vi "Project-overflow.vi"() -> ()   [LabVIEW 2016]
uses:
  <vilib>/DAQmx/read.llb/DAQmx Read (Digital Bool 1Line 1Point).vi
  <vilib>/DAQmx/create/channels.llb/DAQmx Create Channel (DI-Digital Input).vi
  <vilib>/DAQmx/write.llb/DAQmx Write (Digital Bool 1Line 1Point).vi
  <vilib>/DAQmx/create/channels.llb/DAQmx Create Channel (DO-Digital Output).vi
  <vilib>/ptbypt/NI_PtbyPt.lvlib
panel:
  out "Laser Sensor":bool
  in  "Emergency Stop":bool
  out "Use R2":bool
  out "Use R1":bool
  out "Register Bit #1":bool
  out "Register Bit #2":bool
  out "Output Queue Counter":dbl
  out "Rejection Pusher":bool
  out "Metal Sensor 2":bool
  out "Proximity Sensor":bool
  out "Complete or not":bool
  out "Plastic In Queue":dbl
  out "Hopper":bool
  out "Pusher":bool=TRUE
  out "Plastic or not":bool
  out "Belt 2":bool=TRUE
  out "Belt 1":bool=TRUE
  out "Stoped":bool=TRUE
  out "Started":bool=TRUE
  in  "PAUSE":bool
  in  "OFF":bool
  in  "ON":bool
  out "Rejected Pieces":dbl
  out "Completed Pieces":dbl
  out "Don't Push?":bool
  out "Is there anything there?":bool
  # "Main Control"
  # "Sorting Station"
  # "QA Sorting Station"
  # "QA Sorting Register Value"
  # "Result Counter"
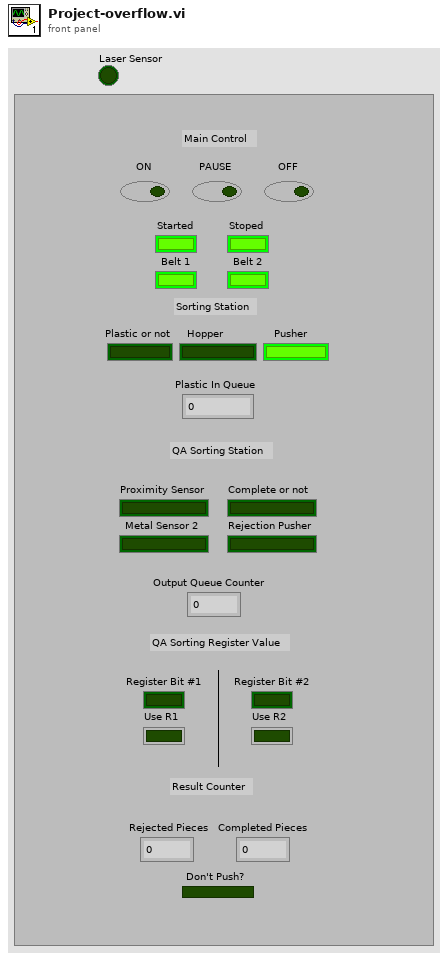
[diagram p1: front panel]
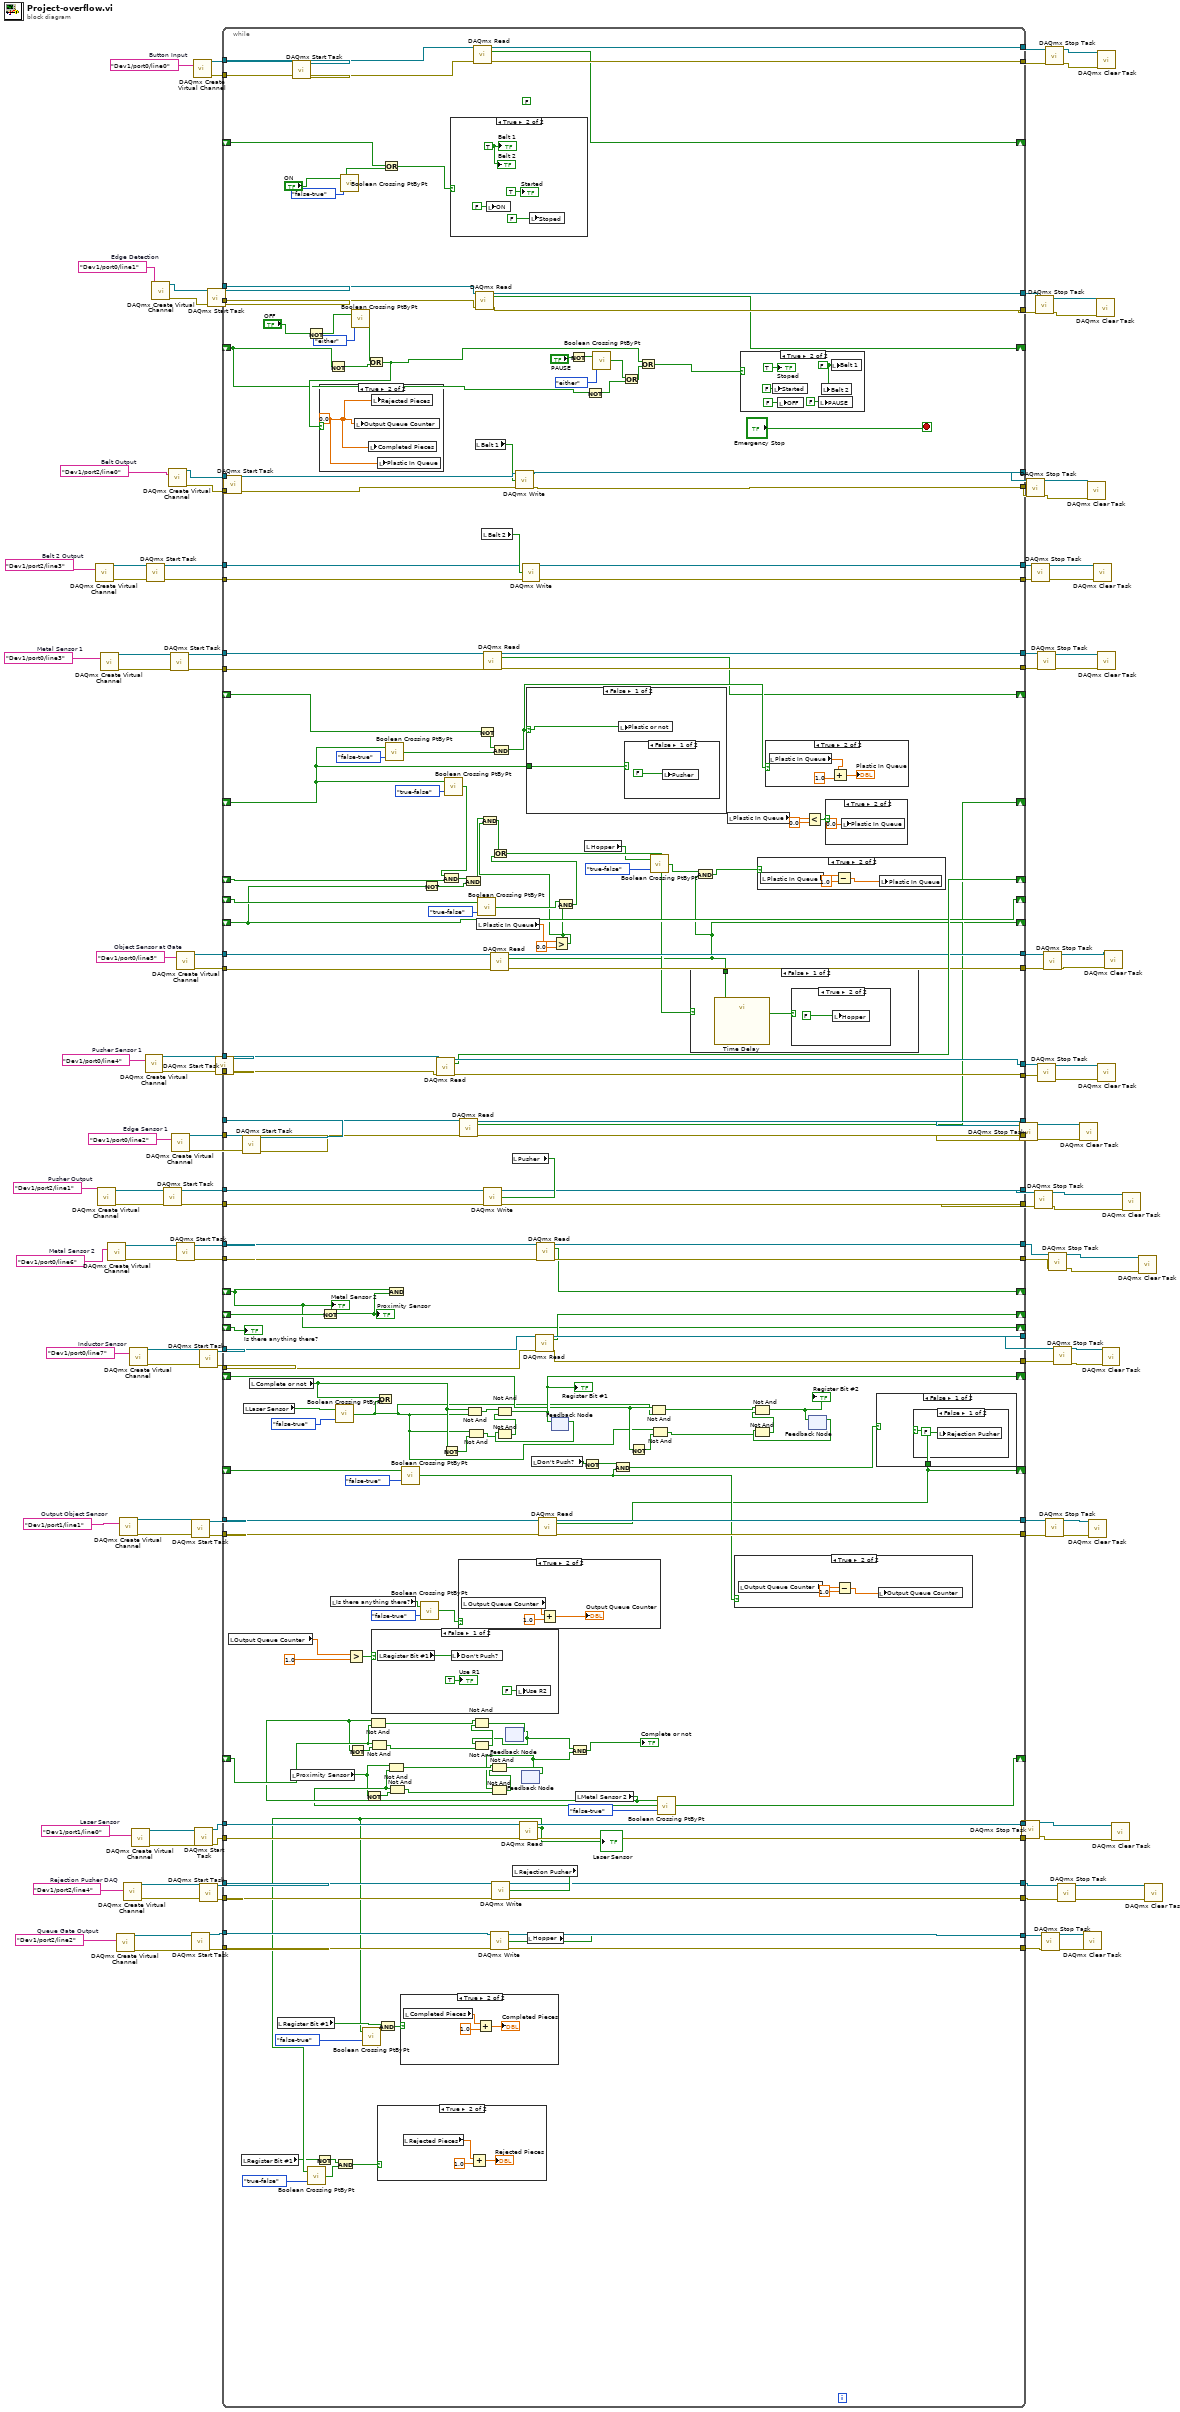
[diagram p0: block diagram]
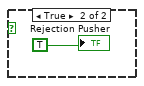
[diagram p3: hidden frame]
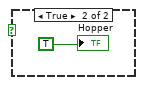
[diagram p5: hidden frame]
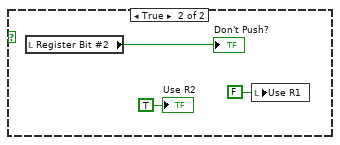
[diagram p12: hidden frame]
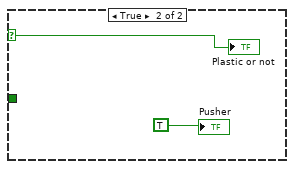
[diagram p16: hidden frame]
diagram:
  w5 = tag "Dev1/port0/line5"  # Object Sensor at Gate
  w12 = tag "Dev1/port1/line0"  # Laser Sensor
  w25 = tag "Dev1/port0/line7"  # Inductor Sensor
  w28 = tag "Dev1/port1/line1"  # Output Object Sensor
  w43 = tag "Dev1/port0/line6"  # Metal Sensor 2
  w46 = tag "Dev1/port2/line4"  # Rejection Pusher DAQ
  w57 = tag "Dev1/port2/line2"  # Queue Gate Output
  w64 = tag "Dev1/port2/line3"  # Belt 2 Output
  w75 = tag "Dev1/port0/line4"  # Pusher Sensor 1
  w84 = tag "Dev1/port0/line2"  # Edge Sensor 1
  w89 = tag "Dev1/port2/line1"  # Pusher Output
  w90 = tag "Dev1/port0/line1"  # Edge Detection
  w91 = tag "Dev1/port0/line0"  # Button Input
  w92 = tag "Dev1/port0/line3"  # Metal Sensor 1
  w93 = tag "Dev1/port2/line0"  # Belt Output
  n1 = call-poly <vilib>:"DAQmx Create Virtual Channel.vi"("lines"=w64) -> ("task out"=w66:refnum<k21>, "error out"=w65:errorcluster)  [unwired: 13 in]
  n2 = call-poly <vilib>:"DAQmx Create Virtual Channel.vi"("lines"=w89) -> ("task out"=w101:refnum<k21>, "error out"=w100:errorcluster)  [unwired: 13 in]
  n3 = call-poly <vilib>:"DAQmx Create Virtual Channel.vi"("lines"=w92) -> ("task out"=w109:refnum<k21>, "error out"=w108:errorcluster)  [unwired: 13 in]
  n4 = call-poly <vilib>:"DAQmx Create Virtual Channel.vi"("lines"=w43) -> ("task out"=w45:refnum<k21>, "error out"=w44:errorcluster)  [unwired: 13 in]
  n5 = call-poly <vilib>:"DAQmx Create Virtual Channel.vi"("lines"=w57) -> ("task out"=w59:refnum<k21>, "error out"=w58:errorcluster)  [unwired: 13 in]
  n6 = call-poly <vilib>:"DAQmx Create Virtual Channel.vi"("lines"=w28) -> ("task out"=w30:refnum<k21>, "error out"=w29:errorcluster)  [unwired: 13 in]
  n7 = call-poly <vilib>:"DAQmx Create Virtual Channel.vi"("lines"=w46) -> ("task out"=w48:refnum<k21>, "error out"=w47:errorcluster)  [unwired: 13 in]
  n8 = call-poly <vilib>:"DAQmx Create Virtual Channel.vi"("lines"=w25) -> ("task out"=w27:refnum<k21>, "error out"=w26:errorcluster)  [unwired: 13 in]
  n9 = call-poly <vilib>:"DAQmx Create Virtual Channel.vi"("lines"=w12) -> ("task out"=w14:refnum<k21>, "error out"=w13:errorcluster)  [unwired: 13 in]
  n10 = call-poly <vilib>:"DAQmx Create Virtual Channel.vi"("lines"=w75) -> ("task out"=w77:refnum<k21>, "error out"=w76:errorcluster)  [unwired: 13 in]
  n11 = call <vilib>:"DAQmx Start Task.vi"("task/channels in"=w66, "error in"=w65) -> ("task out"=w63:refnum<k21>, "error out"=w62:errorcluster)  [unwired: 12 in]
  n12 = call-poly <vilib>:"DAQmx Create Virtual Channel.vi"("lines"=w90) -> ("task out"=w125:refnum<k21>, "error out"=w124:errorcluster)  [unwired: 13 in]
  n13 = call <vilib>:"DAQmx Start Task.vi"("task/channels in"=w101, "error in"=w100) -> ("task out"=w95:refnum<k21>, "error out"=w94:errorcluster)  [unwired: 12 in]
  n14 = call-poly <vilib>:"DAQmx Create Virtual Channel.vi"("lines"=w93) -> ("task out"=w113:refnum<k21>, "error out"=w112:errorcluster)  [unwired: 13 in]
  n15 = call <vilib>:"DAQmx Start Task.vi"("task/channels in"=w109, "error in"=w108) -> ("task out"=w107:refnum<k21>, "error out"=w106:errorcluster)  [unwired: 12 in]
  n16 = call-poly <vilib>:"DAQmx Create Virtual Channel.vi"("lines"=w84) -> ("task out"=w86:refnum<k21>, "error out"=w85:errorcluster)  [unwired: 13 in]
  n17 = call <vilib>:"DAQmx Start Task.vi"("task/channels in"=w45, "error in"=w44) -> ("task out"=w40:refnum<k21>, "error out"=w39:errorcluster)  [unwired: 12 in]
  n18 = call-poly <vilib>:"DAQmx Create Virtual Channel.vi"("lines"=w5) -> ("task out"=w4:refnum<k21>, "error out"=w3:errorcluster)  [unwired: 13 in]
  n19 = call <vilib>:"DAQmx Start Task.vi"("task/channels in"=w30, "error in"=w29) -> ("task out"=w24:refnum<k21>, "error out"=w23:errorcluster)  [unwired: 12 in]
  n20 = call <vilib>:"DAQmx Start Task.vi"("task/channels in"=w59, "error in"=w58) -> ("task out"=w56:refnum<k21>, "error out"=w55:errorcluster)  [unwired: 12 in]
  n21 = call-poly <vilib>:"DAQmx Create Virtual Channel.vi"("lines"=w91) -> ("task out"=w133:refnum<k21>, "error out"=w132:errorcluster)  [unwired: 13 in]
  n22 = call <vilib>:"DAQmx Start Task.vi"("task/channels in"=w14, "error in"=w13) -> ("task out"=w11:refnum<k21>, "error out"=w8:errorcluster)  [unwired: 12 in]
  n23 = call <vilib>:"DAQmx Start Task.vi"("task/channels in"=w27, "error in"=w26) -> ("task out"=w22:refnum<k21>, "error out"=w21:errorcluster)  [unwired: 12 in]
  n24 = call <vilib>:"DAQmx Start Task.vi"("task/channels in"=w48, "error in"=w47) -> ("task out"=w38:refnum<k21>, "error out"=w37:errorcluster)  [unwired: 12 in]
  n25 = call <vilib>:"DAQmx Start Task.vi"("task/channels in"=w125, "error in"=w124) -> ("task out"=w122:refnum<k21>, "error out"=w123:errorcluster)  [unwired: 12 in]
  n26 = call <vilib>:"DAQmx Start Task.vi"("task/channels in"=w77, "error in"=w76) -> ("task out"=w74:refnum<k21>, "error out"=w73:errorcluster)  [unwired: 12 in]
  n27 = call <vilib>:"DAQmx Start Task.vi"("task/channels in"=w113, "error in"=w112) -> ("task out"=w111:refnum<k21>, "error out"=w110:errorcluster)  [unwired: 12 in]
  n28 = call <vilib>:"DAQmx Start Task.vi"("task/channels in"=w86, "error in"=w85) -> ("task out"=w83:refnum<k21>, "error out"=w82:errorcluster)  [unwired: 12 in]
  n29 = call <vilib>:"DAQmx Start Task.vi"("task/channels in"=w133, "error in"=w132) -> ("task out"=w131:refnum<k21>, "error out"=w130:errorcluster)  [unwired: 12 in]
  n30 = while {
    tunnel: w131 -> [w317]
    tunnel: w130 -> [w316]
    tunnel: [w315] -> w129
    tunnel: [w314] -> w128
    shift-right: [w312] -> _
    shift-left: _ -> [w246]
    tunnel: w123 -> [w311]
    tunnel: w122 -> [w310]
    tunnel: [w309] -> w121
    tunnel: [w308] -> w118
    shift-right: [w307] -> _
    shift-left: _ -> [w184]
    tunnel: [w306] -> w115
    tunnel: [w303] -> w114
    tunnel: w111 -> [w305]
    tunnel: w110 -> [w304]
    tunnel: w107 -> [w301]
    tunnel: w106 -> [w300]
    tunnel: [w299] -> w103
    tunnel: [w298] -> w102
    shift-right: [w157] -> _
    shift-left: _ -> [w156]
    tunnel: [w296] -> w97
    tunnel: [w295] -> w96
    tunnel: w95 -> [w294]
    tunnel: w94 -> [w293]
    tunnel: w83 -> [w292]
    tunnel: w82 -> [w291]
    tunnel: [w290] -> w81
    tunnel: [w289] -> w80
    shift-right: [w159] -> _
    shift-left: _ -> [w152]
    tunnel: w74 -> [w287]
    tunnel: w73 -> [w286]
    tunnel: [w285] -> w72
    tunnel: [w284] -> w71
    tunnel: [w281] -> w68
    tunnel: [w280] -> w67
    tunnel: w63 -> [w279]
    tunnel: w62 -> [w278]
    tunnel: w56 -> [w277]
    tunnel: w55 -> [w276]
    tunnel: [w275] -> w54
    tunnel: [w274] -> w53
    shift-right: [w272] -> _
    shift-left: _ -> [w271]
    tunnel: [w267] -> w42
    tunnel: [w266] -> w41
    tunnel: w40 -> [w265]
    tunnel: w39 -> [w264]
    tunnel: w38 -> [w263]
    tunnel: w37 -> [w262]
    tunnel: [w261] -> w36
    tunnel: [w260] -> w35
    shift-right: [w259] -> _
    shift-left: _ -> [w212]
    tunnel: w24 -> [w258]
    tunnel: w23 -> [w257]
    tunnel: w22 -> [w256]
    tunnel: w21 -> [w255]
    tunnel: [w254] -> w20
    tunnel: [w253] -> w19
    tunnel: [w252] -> w18
    tunnel: [w251] -> w17
    shift-right: [w160] -> _
    shift-left: _ -> [w234]
    shift-right: [w250] -> _
    shift-left: _ -> [w249]
    shift-right: [w212] -> _
    shift-left: _ -> [w236]
    tunnel: w11 -> [w232]
    tunnel: [w231] -> w10
    tunnel: [w230] -> w9
    tunnel: w8 -> [w229]
    shift-right: [w214] -> _
    shift-left: _ -> [w213]
    tunnel: w4 -> [w183]
    tunnel: w3 -> [w182]
    tunnel: [w181] -> w2
    tunnel: [w180] -> w1
    shift-right: [w154] -> _
    shift-left: _ -> [w175]
    shift-right: [w175] -> _
    shift-left: _ -> [w178]
    shift-right: [w138] -> _
    shift-left: _ -> [w145]
    stop <- "Emergency Stop" stop-if-true
    (unwired) FALSE ("Boolean")
    n31 = local read "Output Queue Counter"() -> (w222:dbl)
    n32 = local read "Register Bit #1"() -> (w193:bool)
    n33 = local read "Laser Sensor"() -> (w237:bool)
    n34 = local read "Complete or not"() -> (w211:bool)
    n35 = local read "Register Bit #1"() -> (w200:bool)
    n36 = local read "Proximity Sensor"() -> (w137:bool)
    n37 = Not(x="OFF") -> (.not. x?=w206:bool)
    n38 = Not(x=w193) -> (.not. x?=w194:bool)
    n39 = Not(x=w249) -> (.not. x?=w244:bool)
    "Proximity Sensor" <- w244
    n40 = Not(x=w184) -> (.not. x?=w245:bool)
    n41 = local read "Is there anything there?"() -> (w226:bool)
    n42 = call <vilib>:"Boolean Crossing PtByPt.vi"("direction"=enum16{"either", "false-true", "true-false"}."false-true", "input"=w237) -> ("crossing"=w210:bool)  [unwired: 1 in]
    n43 = call <vilib>:"Boolean Crossing PtByPt.vi"("direction"=enum16{"either", "false-true", "true-false"}."false-true", "input"="ON") -> ("crossing"=w209:bool)  [unwired: 1 in]
    n44 = Greater?(x=w222, y=1.0) -> (0:w221:bool)
    n45 = call <vilib>:"Boolean Crossing PtByPt.vi"("direction"=enum16{"either", "false-true", "true-false"}."either", "input"=w206) -> ("crossing"=w207:bool)  [unwired: 1 in]
    n46 = Not(x=w137) -> (.not. x?=w140:bool)
    n47 = Or(x=w207, y=w245) -> (x .or. y?=w185:bool)
    n48 = case shown="True" w185 {
      frame False {
      }
      frame True {
        w331 = 0.0 ("Completed Piece")
        n49 = local write "Output Queue Counter"(w331) -> ()
        n50 = local write "Completed Pieces"(w331) -> ()
        n51 = local write "Rejected Pieces"(w331) -> ()
        n52 = local write "Plastic In Queue"(w331) -> ()
      }
    }
    n53 = case shown="False" w221 {
      frame False {
        n54 = local read "Register Bit #1"() -> (w340:bool)
        n55 = local write "Don't Push?"(w340) -> ()
        n56 = local write "Use R2"(FALSE ("Use R2")) -> ()
        "Use R1" <- TRUE ("Use R1")
      }
      frame True {
        n57 = local read "Register Bit #2"() -> (→"Don't Push?":bool)
        n58 = local write "Use R1"(FALSE ("Use R1")) -> ()
        "Use R2" <- TRUE ("Use R2")
      }
    }
    n59 = Or(x=w211, y=w210) -> ()  [unwired: 1 out]
    n60 = Or(x=w246, y=w209) -> (x .or. y?=w247:bool)
    n61 = call <vilib>:"Boolean Crossing PtByPt.vi"("direction"=enum16{"either", "false-true", "true-false"}."false-true", "input"=w152) -> ("crossing"=w273:bool)  [unwired: 1 in]
    n62 = And(x=w212, y=w244) -> ()  [unwired: 1 out]
    n63 = call <vilib>:"Boolean Crossing PtByPt.vi"("direction"=enum16{"either", "false-true", "true-false"}."false-true", "input"=w234) -> ("crossing"=w224:bool)  [unwired: 1 in]
    n64 = call <vilib>:"Boolean Crossing PtByPt.vi"("direction"=enum16{"either", "false-true", "true-false"}."false-true", "input"=w226) -> ("crossing"=w227:bool)  [unwired: 1 in]
    n65 = Not(x=w175) -> (.not. x?=w176:bool)
    n66 = call-poly <vilib>:"DAQmx Read.vi"("task/channels in"=w287, "error in"=w286) -> ("task out"=w284:refnum<k21>, "data"=w272:bool, "error out"=w285:errorcluster)  [unwired: 11 in]
    n67 = Not(x=w211) -> (.not. x?=w239:bool)
    n68 = call <vilib>:"Boolean Crossing PtByPt.vi"("direction"=enum16{"either", "false-true", "true-false"}."true-false", "input"=w152) -> ("crossing"=w269:bool)  [unwired: 1 in]
    n69 = And(x=w269, y=w271) -> (x .and. y?=w177:bool)
    n70 = case shown="True" w247 {
      frame False {
      }
      frame True {
        w361 = TRUE
        n71 = local write "ON"(FALSE ("ON")) -> ()
        n72 = local write "Stoped"(FALSE) -> ()
        "Started" <- TRUE ("Boolean")
        "Belt 1" <- w361
        "Belt 2" <- w361
      }
    }
    n73 = case shown="True" w227 {
      frame False {
      }
      frame True {
        n74 = local read "Output Queue Counter"() -> (w347:dbl)
        n75 = Add(x=w347, y=1.0) -> (x+y=→"Output Queue Counter":dbl)
      }
    }
    n76 = call-poly <vilib>:"DAQmx Read.vi"("task/channels in"=w292, "error in"=w291) -> ("task out"=w289:refnum<k21>, "data"=w159:bool, "error out"=w290:errorcluster)  [unwired: 11 in]
    n77 = And(x=w177, y=w176) -> (x .and. y?=w169:bool)
    n78 = Not And(1:w210, 2:w211) -> (0:w240:bool)
    n79 = Not And(1:w239, 2:w210) -> (0:w241:bool)
    n80 = call-poly <vilib>:"DAQmx Read.vi"("task/channels in"=w317, "error in"=w316) -> ("task out"=w315:refnum<k21>, "data"=w312:bool, "error out"=w314:errorcluster)  [unwired: 11 in]
    n81 = call-poly <vilib>:"DAQmx Read.vi"("task/channels in"=w310, "error in"=w311) -> ("task out"=w309:refnum<k21>, "data"=w307:bool, "error out"=w308:errorcluster)  [unwired: 11 in]
    n82 = local read "Belt 1"() -> (w302:bool)
    n83 = local read "Plastic In Queue"() -> (w173:dbl)
    n84 = call <vilib>:"Boolean Crossing PtByPt.vi"("direction"=enum16{"either", "false-true", "true-false"}."true-false", "input"=w178) -> ("crossing"=w171:bool)  [unwired: 1 in]
    n85 = Not(x=w156) -> (.not. x?=w288:bool)
    n86 = local read "Belt 2"() -> (w282:bool)
    n87 = call-poly <vilib>:"DAQmx Read.vi"("task/channels in"=w301, "error in"=w300) -> ("task out"=w299:refnum<k21>, "data"=w157:bool, "error out"=w298:errorcluster)  [unwired: 11 in]
    n88 = call-poly <vilib>:"DAQmx Read.vi"("task/channels in"=w183, "error in"=w182) -> ("task out"=w181:refnum<k21>, "data"=w154:bool, "error out"=w180:errorcluster)  [unwired: 11 in]
    n89 = And(x=w288, y=w273) -> (x .and. y?=w174:bool)
    n90 = feedback #1() -> (w136:bool)  [unwired: 1 in]
    n91 = local read "Pusher"() -> (w297:bool)
    n92 = call-poly <vilib>:"DAQmx Write.vi"("task/channels in"=w294, "data"=w297, "error in"=w293) -> ("task out"=w296:refnum<k21>, "error out"=w295:errorcluster)  [unwired: 10 in, 1 out]
    n93 = local read "Rejection Pusher"() -> (w268:bool)
    n94 = call-poly <vilib>:"DAQmx Write.vi"("task/channels in"=w263, "data"=w268, "error in"=w262) -> ("task out"=w261:refnum<k21>, "error out"=w260:errorcluster)  [unwired: 10 in, 1 out]
    n95 = call-poly <vilib>:"DAQmx Write.vi"("task/channels in"=w305, "data"=w302, "error in"=w304) -> ("task out"=w306:refnum<k21>, "error out"=w303:errorcluster)  [unwired: 10 in, 1 out]
    n96 = call-poly <vilib>:"DAQmx Read.vi"("task/channels in"=w232, "error in"=w229) -> ("task out"=w231:refnum<k21>, "data"=w197:bool, "error out"=w230:errorcluster)  [unwired: 11 in]
    "Laser Sensor" <- w197
    n97 = call <vilib>:"Boolean Crossing PtByPt.vi"("direction"=enum16{"either", "false-true", "true-false"}."true-false", "input"=w197) -> ("crossing"=w195:bool)  [unwired: 1 in]
    n98 = And(x=w194, y=w195) -> (x .and. y?=w196:bool)
    n99 = call <vilib>:"Boolean Crossing PtByPt.vi"("direction"=enum16{"either", "false-true", "true-false"}."false-true", "input"=w197) -> ("crossing"=w199:bool)  [unwired: 1 in]
    n100 = case shown="True" w196 {
      frame False {
      }
      frame True {
        n101 = local read "Rejected Pieces"() -> (w333:dbl)
        n102 = Add(x=w333, y=1.0) -> (x+y=→"Rejected Pieces":dbl)
      }
    }
    n103 = And(x=w200, y=w199) -> (x .and. y?=w198:bool)
    n104 = case shown="True" w198 {
      frame False {
      }
      frame True {
        n105 = local read "Completed Pieces"() -> (w335:dbl)
        n106 = Add(x=w335, y=1.0) -> (x+y=→"Completed Pieces":dbl)
      }
    }
    n107 = feedback #2() -> (w135:bool)  [unwired: 1 in]
    n108 = call-poly <vilib>:"DAQmx Write.vi"("task/channels in"=w279, "data"=w282, "error in"=w278) -> ("task out"=w281:refnum<k21>, "error out"=w280:errorcluster)  [unwired: 10 in, 1 out]
    n109 = case shown="False" w174 {
      selector: w174 -> [w351 w354]
      tunnel: w152 -> [w350 _]
      frame False {
        n110 = local write "Plastic or not"(w351) -> ()
        n111 = case shown="False" w350 {
          frame False {
            n112 = local write "Pusher"(FALSE) -> ()
          }
          frame True {
          }
        }
      }
      frame True {
        "Plastic or not" <- w354
        "Pusher" <- TRUE
      }
    }
    n113 = local read "Hopper"() -> (w248:bool)
    n114 = call-poly <vilib>:"DAQmx Write.vi"("task/channels in"=w277, "data"=w248, "error in"=w276) -> ("task out"=w275:refnum<k21>, "error out"=w274:errorcluster)  [unwired: 10 in, 1 out]
    n115 = local read "Don't Push?"() -> (w228:bool)
    n116 = call-poly <vilib>:"DAQmx Read.vi"("task/channels in"=w256, "error in"=w255) -> ("task out"=w251:refnum<k21>, "data"=w250:bool, "error out"=w252:errorcluster)  [unwired: 11 in]
    n117 = call-poly <vilib>:"DAQmx Read.vi"("task/channels in"=w265, "error in"=w264) -> ("task out"=w267:refnum<k21>, "data"=w259:bool, "error out"=w266:errorcluster)  [unwired: 11 in]
    n118 = call-poly <vilib>:"DAQmx Read.vi"("task/channels in"=w258, "error in"=w257) -> ("task out"=w254:refnum<k21>, "data"=w160:bool, "error out"=w253:errorcluster)  [unwired: 11 in]
    n119 = feedback #3() -> (w242:bool)  [unwired: 1 in]
    n120 = Not And(1:w241, 2:w242) -> (0:w243:bool)
    n121 = Not And(1:w243, 2:w240) -> (0:w214:bool)
    "Register Bit #1" <- w214
    n122 = feedback-in #3(w214) -> ()
    n123 = Greater?(x=w173, y=0.0) -> (0:w168:bool)
    n124 = And(x=w169, y=w168) -> (x .and. y?=w164:bool)
    n125 = And(x=w171, y=w168) -> (x .and. y?=w163:bool)
    n126 = Or(x=w164, y=w163) -> (x .or. y?=w162:bool)
    n127 = Not(x="PAUSE") -> (.not. x?=w190:bool)
    n128 = And(x=w136, y=w135) -> (x .and. y?=→"Complete or not":bool)
    n129 = local read "Metal Sensor 2"() -> (w144:bool)
    n130 = Not(x=w144) -> (.not. x?=w148:bool)
    n131 = Not And(1:w145, 2:w144) -> (0:w149:bool)
    n132 = Not And(1:w148, 2:w145) -> (0:w150:bool)
    n133 = Not And(1:w150, 2:w136) -> (0:w151:bool)
    n134 = Not And(1:w151, 2:w149) -> (0:w147:bool)
    n135 = feedback-in #1(w147) -> ()
    n136 = Not(x=w228) -> (.not. x?=w235:bool)
    n137 = local read "Hopper"() -> (w158:bool)
    n138 = Not(x=w184) -> (.not. x?=w192:bool)
    n139 = call <vilib>:"Boolean Crossing PtByPt.vi"("direction"=enum16{"either", "false-true", "true-false"}."either", "input"=w190) -> ("crossing"=w191:bool)  [unwired: 1 in]
    n140 = And(x=w235, y=w224) -> (x .and. y?=w161:bool)
    n141 = Or(x=w191, y=w192) -> (x .or. y?=w186:bool)
    n142 = Not(x=w213) -> (.not. x?=w216:bool)
    n143 = Or(x=w185, y=w186) -> (x .or. y?=w187:bool)
    n144 = call <vilib>:"Boolean Crossing PtByPt.vi"("direction"=enum16{"either", "false-true", "true-false"}."true-false", "input"=w158) -> ("crossing"=w155:bool)  [unwired: 1 in]
    n145 = Not And(1:w210, 2:w213) -> (0:w217:bool)
    n146 = Not And(1:w216, 2:w210) -> (0:w218:bool)
    n147 = call <vilib>:"Boolean Crossing PtByPt.vi"("direction"=enum16{"either", "false-true", "true-false"}."false-true", "input"=w144) -> ("crossing"=w138:bool)  [unwired: 1 in]
    n148 = Not And(1:w138, 2:w137) -> (0:w141:bool)
    n149 = Not And(1:w140, 2:w138) -> (0:w142:bool)
    n150 = Not And(1:w142, 2:w135) -> (0:w143:bool)
    n151 = Not And(1:w143, 2:w141) -> (0:w139:bool)
    n152 = feedback-in #2(w139) -> ()
    n153 = case shown="False" w162 {
      tunnel: w154 -> [w321 _]
      frame False {
        n154 = call "Time Delay"() -> ()  [unwired: 11 in, 1 out]
        n155 = case shown="True" w321 {
          frame False {
          }
          frame True {
            n156 = local write "Hopper"(FALSE) -> ()
          }
        }
      }
      frame True {
        "Hopper" <- TRUE
      }
    }
    n157 = And(x=w155, y=w154) -> (x .and. y?=w153:bool)
    n158 = local read "Plastic In Queue"() -> (w167:dbl)
    n159 = case shown="True" w224 {
      frame False {
      }
      frame True {
        n160 = local read "Output Queue Counter"() -> (w346:dbl)
        n161 = Subtract(x=w346, y=1.0) -> (x-y=w344:dbl)
        n162 = local write "Output Queue Counter"(w344) -> ()
      }
    }
    n163 = case shown="True" w187 {
      frame False {
      }
      frame True {
        w357 = FALSE
        n164 = local write "Started"(FALSE ("Stop")) -> ()
        n165 = local write "OFF"(FALSE ("OFF")) -> ()
        n166 = local write "PAUSE"(FALSE ("Pause")) -> ()
        n167 = local write "Belt 2"(w357) -> ()
        n168 = local write "Belt 1"(w357) -> ()
        "Stoped" <- TRUE
      }
    }
    n169 = case shown="True" w153 {
      frame False {
      }
      frame True {
        n170 = local read "Plastic In Queue"() -> (w326:dbl)
        n171 = Subtract(x=w326, y=1.0) -> (x-y=w327:dbl)
        n172 = local write "Plastic In Queue"(w327) -> ()
      }
    }
    n173 = case shown="True" w174 {
      frame False {
      }
      frame True {
        n174 = local read "Plastic In Queue"() -> (w328:dbl)
        n175 = Add(x=w328, y=1.0) -> (x+y=→"Plastic In Queue":dbl)
      }
    }
    n176 = Less?(x=w167, y=0.0) -> (x < y?=w165:bool)
    n177 = feedback #4() -> (w219:bool)  [unwired: 1 in]
    n178 = Not And(1:w218, 2:w219) -> (0:w220:bool)
    n179 = Not And(1:w220, 2:w217) -> (0:w215:bool)
    "Register Bit #2" <- w215
    n180 = feedback-in #4(w215) -> ()
    n181 = case shown="True" w165 {
      frame False {
      }
      frame True {
        n182 = local write "Plastic In Queue"(0.0 ("Plastic In Queue")) -> ()
      }
    }
    n183 = case shown="False" w161 {
      tunnel: w160 -> [w318 _]
      frame False {
        n184 = case shown="False" w318 {
          frame False {
            n185 = local write "Rejection Pusher"(FALSE) -> ()
          }
          frame True {
          }
        }
      }
      frame True {
        "Rejection Pusher" <- TRUE
      }
    }
    "Metal Sensor 2" <- w212
    "Is there anything there?" <- w236
  }
  n186 = call <vilib>:"DAQmx Stop Task.vi"("task/channels in"=w80, "error in"=w81) -> ("task out"=w88:refnum<k21>, "error out"=w87:errorcluster)  [unwired: 12 in]
  n187 = call <vilib>:"DAQmx Stop Task.vi"("task/channels in"=w10, "error in"=w9) -> ("task out"=w16:refnum<k21>, "error out"=w15:errorcluster)  [unwired: 12 in]
  n188 = call <vilib>:"DAQmx Stop Task.vi"("task/channels in"=w115, "error in"=w114) -> ("task out"=w117:refnum<k21>, "error out"=w116:errorcluster)  [unwired: 12 in]
  n189 = call <vilib>:"DAQmx Stop Task.vi"("task/channels in"=w68, "error in"=w67) -> ("task out"=w70:refnum<k21>, "error out"=w69:errorcluster)  [unwired: 12 in]
  n190 = call <vilib>:"DAQmx Stop Task.vi"("task/channels in"=w97, "error in"=w96) -> ("task out"=w99:refnum<k21>, "error out"=w98:errorcluster)  [unwired: 12 in]
  n191 = call <vilib>:"DAQmx Stop Task.vi"("task/channels in"=w121, "error in"=w118) -> ("task out"=w120:refnum<k21>, "error out"=w119:errorcluster)  [unwired: 12 in]
  n192 = call <vilib>:"DAQmx Stop Task.vi"("task/channels in"=w103, "error in"=w102) -> ("task out"=w105:refnum<k21>, "error out"=w104:errorcluster)  [unwired: 12 in]
  n193 = call <vilib>:"DAQmx Stop Task.vi"("task/channels in"=w71, "error in"=w72) -> ("task out"=w79:refnum<k21>, "error out"=w78:errorcluster)  [unwired: 12 in]
  n194 = call <vilib>:"DAQmx Stop Task.vi"("task/channels in"=w54, "error in"=w53) -> ("task out"=w61:refnum<k21>, "error out"=w60:errorcluster)  [unwired: 12 in]
  n195 = call <vilib>:"DAQmx Stop Task.vi"("task/channels in"=w2, "error in"=w1) -> ("task out"=w7:refnum<k21>, "error out"=w6:errorcluster)  [unwired: 12 in]
  n196 = call <vilib>:"DAQmx Stop Task.vi"("task/channels in"=w20, "error in"=w19) -> ("task out"=w34:refnum<k21>, "error out"=w33:errorcluster)  [unwired: 12 in]
  n197 = call <vilib>:"DAQmx Stop Task.vi"("task/channels in"=w129, "error in"=w128) -> ("task out"=w126:refnum<k21>, "error out"=w127:errorcluster)  [unwired: 12 in]
  n198 = call <vilib>:"DAQmx Stop Task.vi"("task/channels in"=w42, "error in"=w41) -> ("task out"=w50:refnum<k21>, "error out"=w49:errorcluster)  [unwired: 12 in]
  n199 = call <vilib>:"DAQmx Stop Task.vi"("task/channels in"=w17, "error in"=w18) -> ("task out"=w32:refnum<k21>, "error out"=w31:errorcluster)  [unwired: 12 in]
  n200 = call <vilib>:"DAQmx Stop Task.vi"("task/channels in"=w36, "error in"=w35) -> ("task out"=w52:refnum<k21>, "error out"=w51:errorcluster)  [unwired: 12 in]
  n201 = call <vilib>:"DAQmx Clear Task.vi"("task in"=w88, "error in"=w87) -> ()  [unwired: 13 in, 1 out]
  n202 = call <vilib>:"DAQmx Clear Task.vi"("task in"=w61, "error in"=w60) -> ()  [unwired: 13 in, 1 out]
  n203 = call <vilib>:"DAQmx Clear Task.vi"("task in"=w117, "error in"=w116) -> ()  [unwired: 13 in, 1 out]
  n204 = call <vilib>:"DAQmx Clear Task.vi"("task in"=w34, "error in"=w33) -> ()  [unwired: 13 in, 1 out]
  n205 = call <vilib>:"DAQmx Clear Task.vi"("task in"=w70, "error in"=w69) -> ()  [unwired: 13 in, 1 out]
  n206 = call <vilib>:"DAQmx Clear Task.vi"("task in"=w120, "error in"=w119) -> ()  [unwired: 13 in, 1 out]
  n207 = call <vilib>:"DAQmx Clear Task.vi"("task in"=w126, "error in"=w127) -> ()  [unwired: 13 in, 1 out]
  n208 = call <vilib>:"DAQmx Clear Task.vi"("task in"=w105, "error in"=w104) -> ()  [unwired: 13 in, 1 out]
  n209 = call <vilib>:"DAQmx Clear Task.vi"("task in"=w79, "error in"=w78) -> ()  [unwired: 13 in, 1 out]
  n210 = call <vilib>:"DAQmx Clear Task.vi"("task in"=w32, "error in"=w31) -> ()  [unwired: 13 in, 1 out]
  n211 = call <vilib>:"DAQmx Clear Task.vi"("task in"=w7, "error in"=w6) -> ()  [unwired: 13 in, 1 out]
  n212 = call <vilib>:"DAQmx Clear Task.vi"("task in"=w16, "error in"=w15) -> ()  [unwired: 13 in, 1 out]
  n213 = call <vilib>:"DAQmx Clear Task.vi"("task in"=w99, "error in"=w98) -> ()  [unwired: 13 in, 1 out]
  n214 = call <vilib>:"DAQmx Clear Task.vi"("task in"=w50, "error in"=w49) -> ()  [unwired: 13 in, 1 out]
  n215 = call <vilib>:"DAQmx Clear Task.vi"("task in"=w52, "error in"=w51) -> ()  [unwired: 13 in, 1 out]
